vi "Var to Bool（idx）.vi"(2 "Delays":u32, 3 "Error in":errorcluster caption="错误输入", 4 "Var In":variant, 5 "idx":i32) -> (0 "Error out":errorcluster caption="Error in", 1 "Var Out":bool[](array[boolean]))   [LabVIEW 2014]
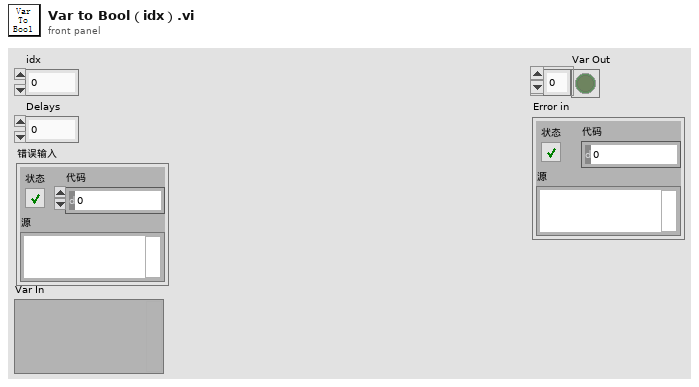
[diagram p1: front panel]
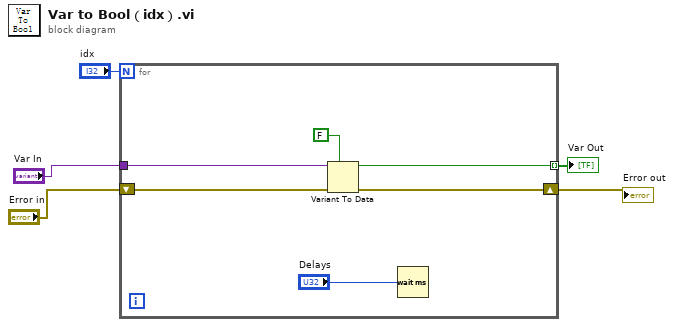
[diagram p0: block diagram]
diagram:
  n1 = for {
    N: "idx" -> [_]
    tunnel: "Var In" -> [w9]
    tunnel: [w8] -> w3 mode=indexing
    shift-right: [w7] -> w1
    shift-left: "Error in" -> [w6]
    n2 = Variant To Data(error in=w6, type=FALSE, Variant=w9) -> (data=w8:bool, error out=w7:errorcluster)
    n3 = Wait (ms)(milliseconds to wait="Delays") -> ()  [unwired: 1 out]
  }
  "Var Out" <- w3
  "Error out" <- w1
